vi "Write State.vi"(8 "error in (no error)":errorcluster, 10 "State":bool, 11 "Change Individual Power Supply MSG in":refnum<class "Change Individual Power Supply MSG.lvclass">) -> (0 "error out":errorcluster, 3 "Change Individual Power Supply MSG out":refnum<class "Change Individual Power Supply MSG.lvclass">)   [LabVIEW 2014, in "Controller.lvlib" / "Change Individual Power Supply MSG.lvclass"]
uses:
  Change Individual Power Supply MSG.lvclass
  Change Individual Power Supply MSG.lvclass/Change Individual Power Supply MSG.ctl
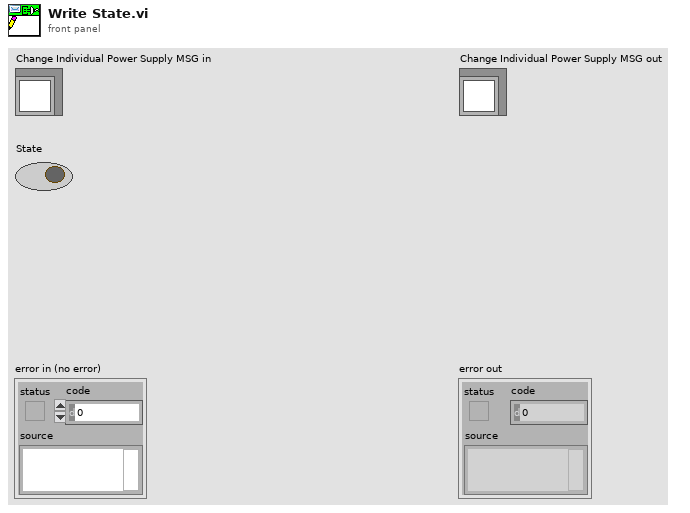
[diagram p1: front panel]
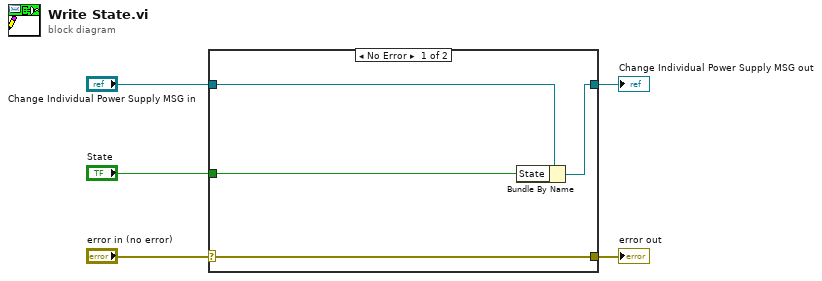
[diagram p0: block diagram]
diagram:
  n1 = case shown="No Error" "error in (no error)" {
    selector: "error in (no error)" -> [w9 w10]
    tunnel: [w9 w10] -> w4
    tunnel: [w7 w11] -> w2
    tunnel: "Change Individual Power Supply MSG in" -> [w8 w11]
    tunnel: "State" -> [w6 _]
    frame No Error {
      n2 = Bundle By Name(cluster=w8, "State"=w6) -> (w7:refnum<class "Change Individual Power Supply MSG.lvclass">)
    }
    frame Error {
    }
  }
  "error out" <- w4
  "Change Individual Power Supply MSG out" <- w2
